vi "Set Tube Parameters.vi"(8 "error in (no error)":errorcluster, 10 "Tube Gas":T1, 11 "Owlstone GEN-SYS in":refnum<class "Owlstone GEN-SYS.lvclass">) -> (0 "error out":errorcluster, 1 "Calibration Temperature":i32, 2 "Permeation Rate":i32, 3 "Owlstone GEN-SYS out":refnum<class "Owlstone GEN-SYS.lvclass">, 4 "Molecular Weight":dbl)   [LabVIEW 2011, in "Owlstone GEN-SYS.lvclass"]
uses:
  Owlstone GEN-SYS.lvclass
  Permeation Tube Gas.ctl
  Owlstone GEN-SYS.lvclass/Owlstone GEN-SYS.ctl
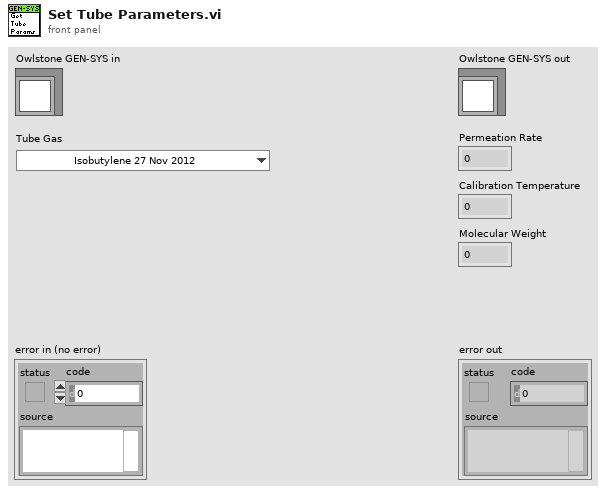
[diagram p1: front panel]
types:
  T1 = typedef "Owlstone GEN-SYS.lvclass/Permeation Tube Gas.ctl" = enum16{"Isobutylene 27 Nov 2012", "Ammonia 29 Sep 2012", "DMMP Tube A 3 July 2014", "DMMP Tube B 3 July 2014"}
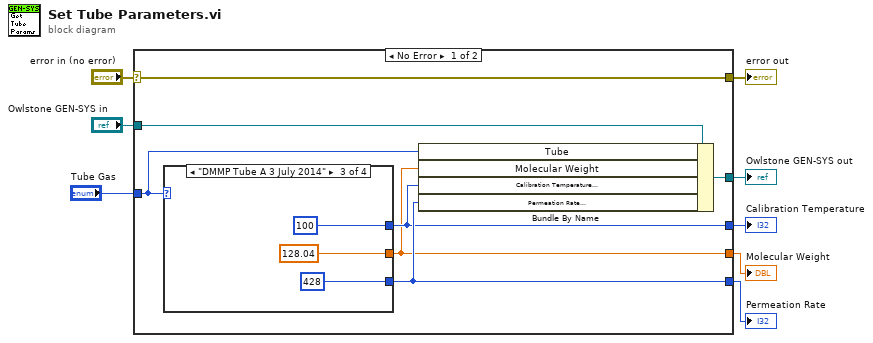
[diagram p0: block diagram]
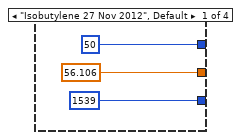
[diagram p2: hidden frame]
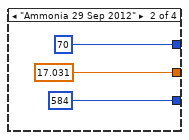
[diagram p3: hidden frame]
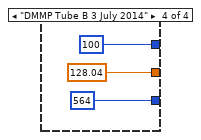
[diagram p4: hidden frame]
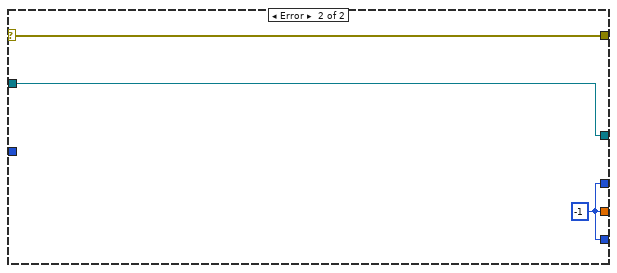
[diagram p5: hidden frame]
diagram:
  n1 = case shown="No Error" "error in (no error)" {
    selector: "error in (no error)" -> [w15 w30]
    tunnel: [w15 w30] -> w7
    tunnel: [w13 w29] -> w5
    tunnel: "Owlstone GEN-SYS in" -> [w14 w29]
    tunnel: "Tube Gas" -> [w12 _]
    tunnel: [w11 w28] -> w4
    tunnel: [w10 w28] -> w3
    tunnel: [w9 w28] -> w2
    frame No Error {
      n2 = case shown="\"DMMP Tube A 3 July 2014\"" w12 {
        tunnel: [56.106 17.031 128.04 128.04] -> w9
        tunnel: [50 70 100 100] -> w10
        tunnel: [1539 584 428 564] -> w11
        frame "Isobutylene 27 Nov 2012", Default {
        }
        frame "Ammonia 29 Sep 2012" {
        }
        frame "DMMP Tube A 3 July 2014" {
        }
        frame "DMMP Tube B 3 July 2014" {
        }
      }
      n3 = Bundle By Name(cluster=w14, "Tube"=w12, "Molecular Weight"=w9, "Calibration Temperature\n(Celcius)"=w10, "Permeation Rate \n(ng/min)"=w11) -> (w13:refnum<class "Owlstone GEN-SYS.lvclass">)
    }
    frame Error {
      w28 = -1
    }
  }
  "error out" <- w7
  "Owlstone GEN-SYS out" <- w5
  "Permeation Rate" <- w4
  "Calibration Temperature" <- w3
  "Molecular Weight" <- w2
